vi "Chi-Squared (Non-Central) Inverse CDF.vi"(9 "d":dbl, 10 "k":i32=1, 11 "cdf(x)":dbl=0.682689492137086) -> (0 "error":i32, 3 "x":dbl=1.0)   [LabVIEW 2017, in "NI_Gmath.lvlib"]
doc: "Computes the continuous inverse cumulative distribution function (CDF) of the various distributions. You must manually select the polymorphic instance to use."
uses:
  <vilib>/gmath/NI_Gmath.lvlib
  <vilib>/gmath/statdist.llb/st_error_code.ctl
panel:
  # "Chi-Squared (Non-Central) \nInverse CDF"
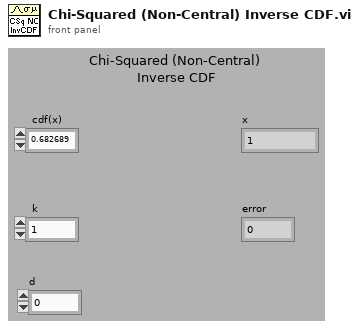
[diagram p1: front panel]
types:
  T1 = typedef "NI_Gmath.lvlib/st_error_code.ctl" = i32
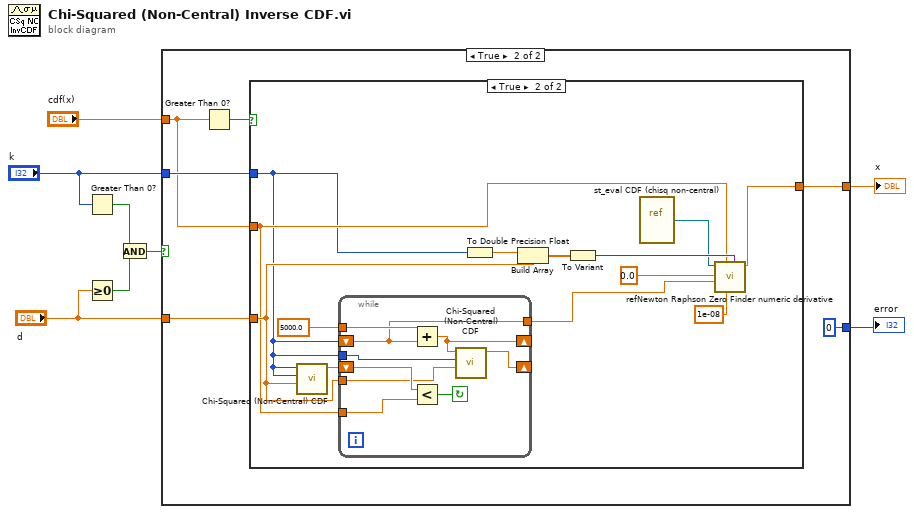
[diagram p0: block diagram]
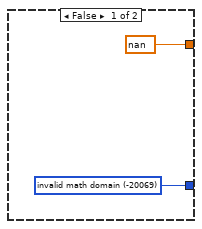
[diagram p2: hidden frame]
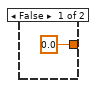
[diagram p3: hidden frame]
diagram:
  n1 = Greater Than 0?(x="k") -> (x > 0?=w4:bool)
  n2 = Greater Or Equal To 0?(x="d") -> (x >= 0?=w5:bool)
  n3 = And(x=w4, y=w5) -> (x .and. y?=w3:bool)
  n4 = case shown="True" w3 {
    tunnel: [w9 0 ("invalid math domain")] -> w8
    tunnel: [nan w15] -> w7
    tunnel: "cdf(x)" -> [_ w13]
    tunnel: "k" -> [_ w14]
    tunnel: "d" -> [_ w11]
    frame False {
      w9 = T1 -20069 items=["invalid math domain"=-20069, "Fourier interpolation size m >= n"=-20070, "empty array"=-20003] ("stat interp error code")
    }
    frame True {
      n5 = Greater Than 0?(x=w13) -> (x > 0?=w12:bool)
      n6 = case shown="True" w12 {
        tunnel: [0.0 w29] -> w15
        tunnel: w13 -> [_ w20]
        tunnel: w14 -> [_ w18]
        tunnel: w11 -> [_ w21]
        frame False {
        }
        frame True {
          n7 = call <vilib>:"Chi-Squared (Non-Central) CDF.vi"("d"=w21, "k"=w18, "x"=w18) -> ("cdf(x)"=w23:dbl)  [unwired: 7 in, 1 out]
          n8 = while {
            shift-right: [w37] -> _
            shift-left: w23 -> [w38]
            shift-right: [w36] -> _
            shift-left: w18 -> [w34]
            tunnel: 5000.0 ("upper limit") -> [w35]
            tunnel: [w34] -> w19
            tunnel: w18 -> [w33]
            tunnel: w21 -> [w32]
            tunnel: w20 -> [w31]
            stop <- w39 continue-if-true
            n9 = Add(x=w35, y=w34) -> (x+y=w36:dbl)
            n10 = Less?(x=w38, y=w31) -> (x < y?=w39:bool)
            n11 = call <vilib>:"Chi-Squared (Non-Central) CDF.vi"("d"=w32, "k"=w33, "x"=w36) -> ("cdf(x)"=w37:dbl)  [unwired: 7 in, 1 out]
          }
          n12 = To Double Precision Float(number=w18) -> (double precision float=w24:dbl)
          n13 = Build Array(w24, w21) -> (w30:dbl[])
          n14 = To Variant(anything=w30) -> (Variant=w28:variant)
          n15 = vi-ref <vilib>:"st_eval CDF (chisq non-central).vi"() -> ("vi reference"=w27:refnum<vi>)
          n16 = call <vilib>:"refNewton Raphson Zero Finder numeric derivative.vi"("function parameters"=w28, "accuracy"=1e-08, "level"=w20, "end"=w19, "start"=0.0 ("upper limit"), "function refnum"=w27) -> ("zero"=w29:dbl)  [unwired: 2 in, 3 out]
        }
      }
    }
  }
  "x" <- w7
  "error" <- w8
